vi "polling acquire doesnt work.vi"(8 "error in (no error)":errorcluster, 10 "ChannelEnable":cluster{"Channel 1":T1, "Channel 2":T1}, 11 "VISA Refnum in":refnum<visa-resource-name>) -> (0 "error out":errorcluster, 1 "Numeric":dbl, 2 "Numeric 2":dbl, 3 "VISA Refnum out":refnum<visa-resource-name>)   [LabVIEW 2020, in "Gentec SlinkUSB.lvclass"]
uses:
  Gentec SlinkUSB.lvclass
  OnOffTypeDef.ctl
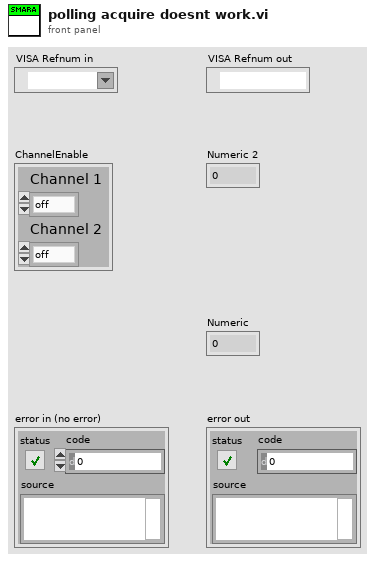
[diagram p1: front panel]
types:
  T1 = typedef "OnOffTypeDef.ctl" = enum16{"off", "on"}
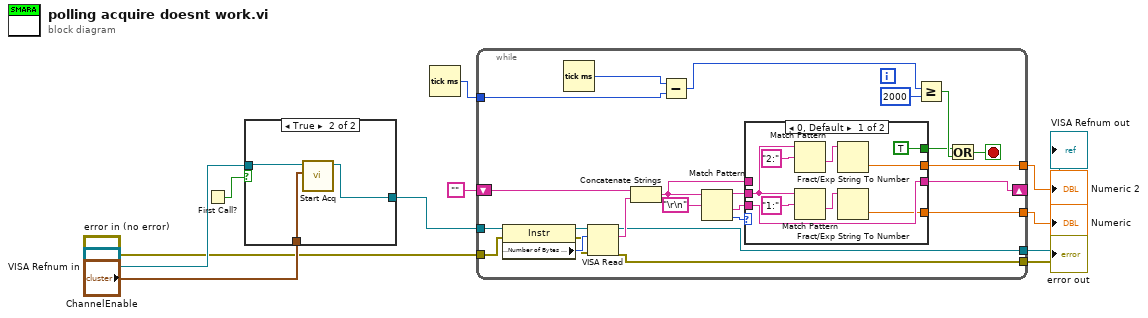
[diagram p0: block diagram]
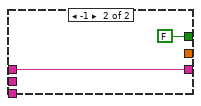
[diagram p3: hidden frame]
diagram:
  n1 = First Call?() -> (First Call?: T/F=w9:bool)
  n2 = case shown="True" w9 {
    tunnel: "VISA Refnum in" -> [w12 w15]
    tunnel: "ChannelEnable" -> [_ w14]
    tunnel: [w12 w13] -> w11
    frame False {
    }
    frame True {
      n3 = call "Start Acq.vi"("ChannelEnable"=w14, "VISA Refnum in"=w15) -> ("VISA Refnum out"=w13:refnum<visa-resource-name>)  [unwired: 8 in, 1 out]
    }
  }
  n4 = Tick Count (ms)() -> (millisecond timer value=w8:u32)
  n5 = while {
    shift-right: [w37] -> _
    shift-left: "" -> [w34]
    tunnel: w11 -> [w32]
    tunnel: [w24] -> w3
    tunnel: [w23] -> w2
    tunnel: [w22] -> w4
    tunnel: [w21] -> w5
    tunnel: "error in (no error)" -> [w19]
    tunnel: w8 -> [w17]
    stop <- w27 stop-if-true
    n6 = property class="Instr"(reference=w32, error in=w19) -> (reference out=w31:refnum<visa-resource-name>, error out=w20:errorcluster, "Serial Settings:Number of Bytes at Serial Port"=w30:u32)
    n7 = Tick Count (ms)() -> (millisecond timer value=w18:u32)
    n8 = VISA Read(VISA resource name=w31, byte count=w30, error in (no error)=w20) -> (VISA resource name out=w22:refnum<visa-resource-name>, read buffer=w25:string, error out=w21:errorcluster)  [unwired: 1 out]
    n9 = Concatenate Strings(w34, w25) -> (w38:string)
    n10 = Subtract(x=w18, y=w17) -> (x-y=w16:u32)
    n11 = Match Pattern(string=w38, regular expression="\r\n") -> (before substring=w35:string, after substring=w36:string, offset past match=w39:i32)  [unwired: 1 in, 1 out]
    n12 = case shown="0, Default" w39 {
      tunnel: [w42 w50] -> w37
      tunnel: w38 -> [_ w50]
      tunnel: w36 -> [w42 _]
      tunnel: w35 -> [w45 _]
      tunnel: [TRUE ("x") FALSE ("x")] -> w28
      tunnel: [w41 _] -> w24
      tunnel: [w40 _] -> w23
      frame 0, Default {
        n13 = Match Pattern(string=w45, regular expression="2:") -> (after substring=w44:string)  [unwired: 1 in, 3 out]
        n14 = Match Pattern(string=w45, regular expression="1:") -> (after substring=w43:string)  [unwired: 1 in, 3 out]
        n15 = Fract/Exp String To Number(string=w44) -> (number=w40:dbl)  [unwired: 3 in, 1 out]
        n16 = Fract/Exp String To Number(string=w43) -> (number=w41:dbl)  [unwired: 3 in, 1 out]
      }
      frame -1 {
      }
    }
    n17 = Greater Or Equal?(x=w16, y=i16 2000 ("x")) -> (x >= y?=w29:bool)
    n18 = Or(x=w28, y=w29) -> (x .or. y?=w27:bool)
  }
  "error out" <- w5
  "VISA Refnum out" <- w4
  "Numeric" <- w3
  "Numeric 2" <- w2
